vi "Movement (SubVI).vi"(4 "Speed":dbl format="%.2f", 5 "Reset":bool, 6 "Acc":dbl format="%.2f", 8 "Goal P":i32, 9 "Goal Y":dbl format="%.2f", 10 "Goal X":dbl format="%.2f") -> (0 "Vp":dbl, 1 "Vy":dbl, 2 "Vx":dbl, 3 "Reach?":bool)   [LabVIEW 2017]
uses:
  Projects/Auto control/Global 1.vi
  Projects/Auto control/Inputs.vi
  Projects/Auto control/Outputs.vi
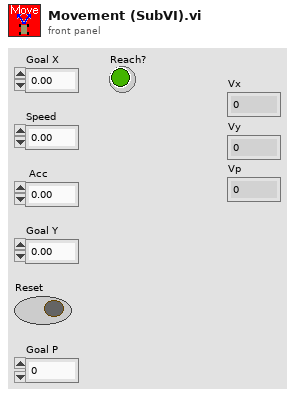
[diagram p1: front panel]
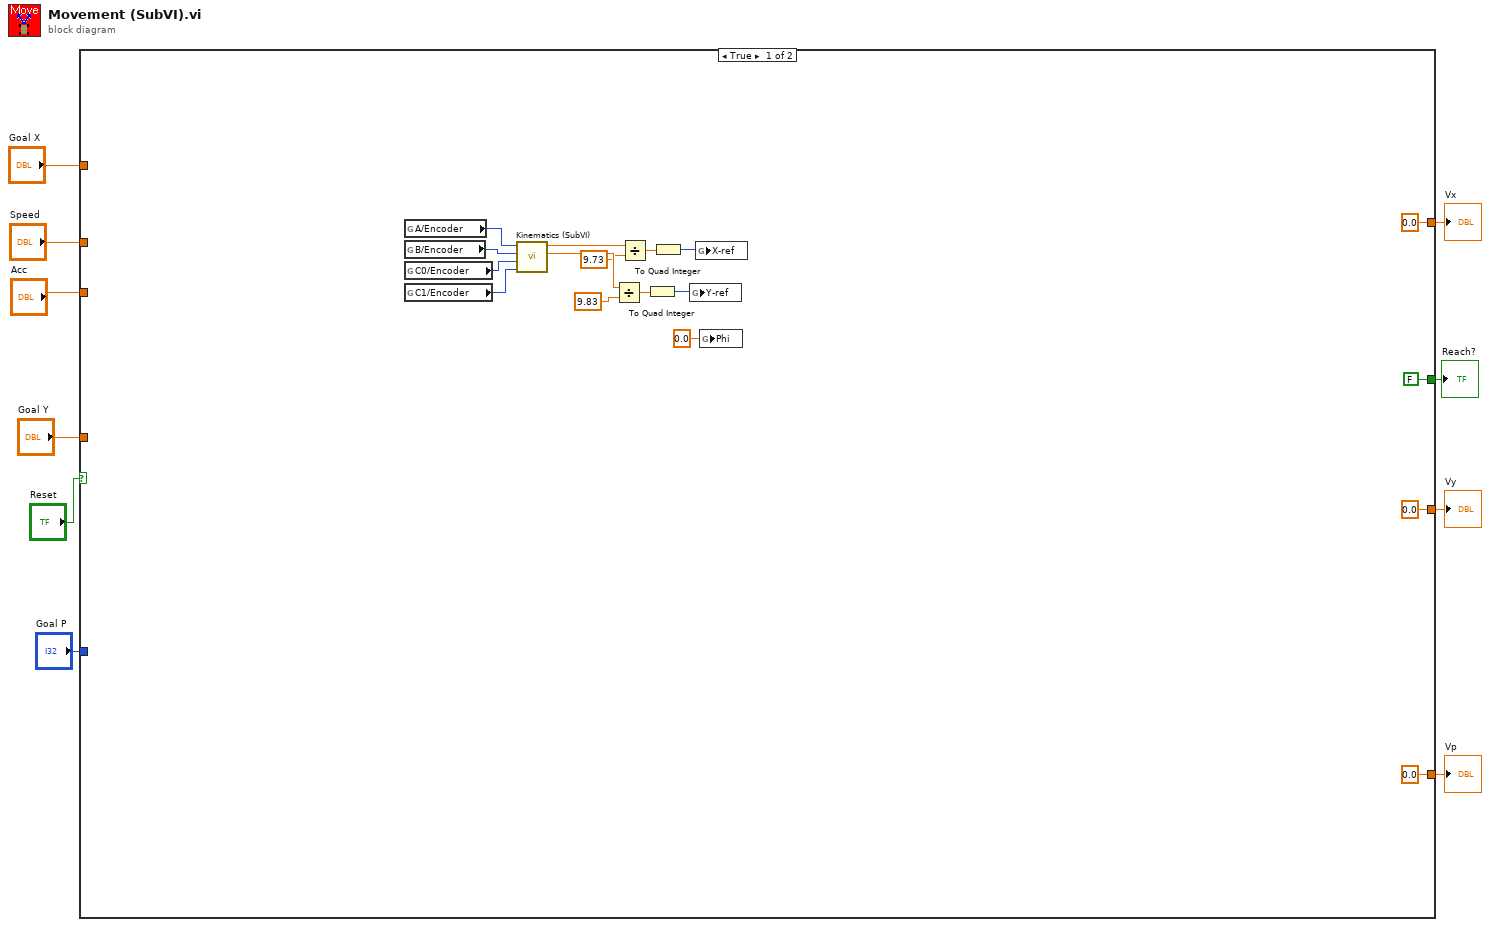
[diagram p0: block diagram]
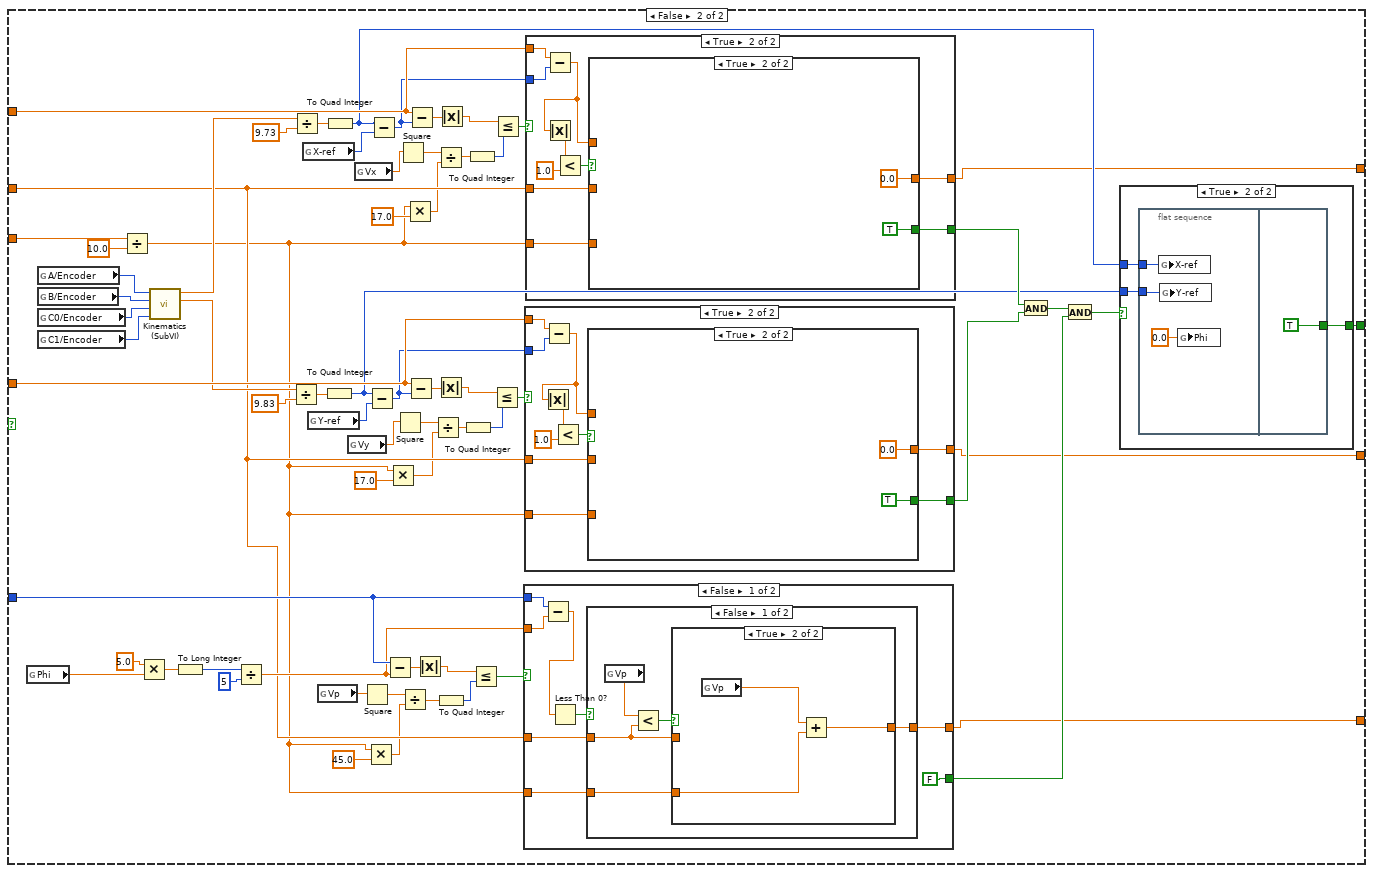
[diagram p2: hidden frame]
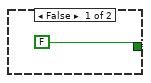
[diagram p3: hidden frame]
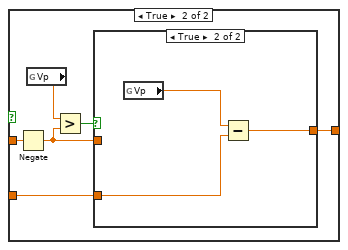
[diagram p5: hidden frame]
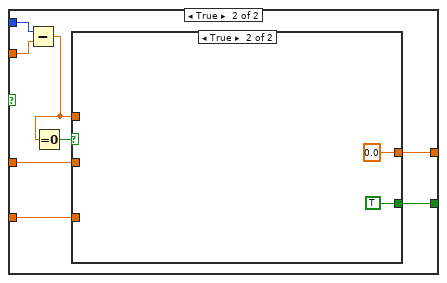
[diagram p7: hidden frame]
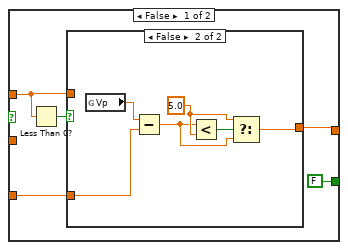
[diagram p8: hidden frame]
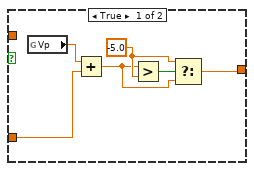
[diagram p9: hidden frame]
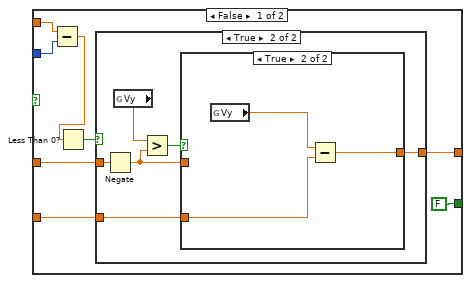
[diagram p10: hidden frame]
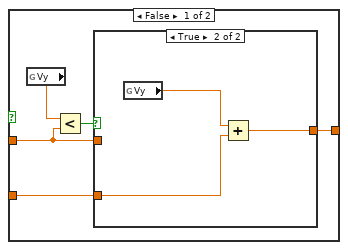
[diagram p11: hidden frame]
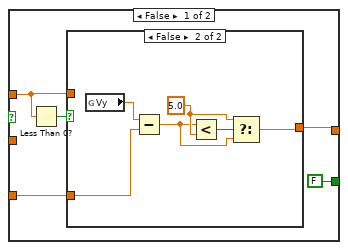
[diagram p14: hidden frame]
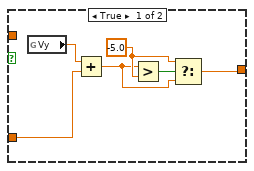
[diagram p15: hidden frame]
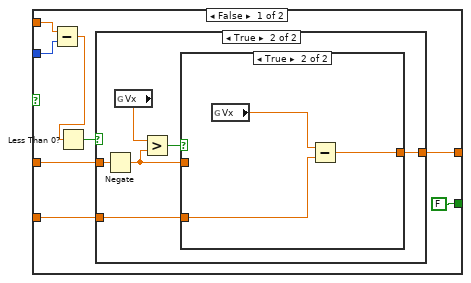
[diagram p16: hidden frame]
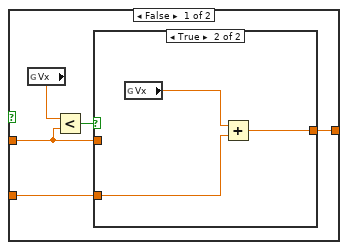
[diagram p17: hidden frame]
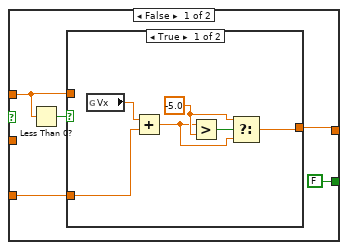
[diagram p20: hidden frame]
diagram:
  n1 = case shown="True" "Reset" {
    tunnel: "Acc" -> [_ w88]
    tunnel: "Goal X" -> [_ w86]
    tunnel: "Goal Y" -> [_ w79]
    tunnel: [FALSE ("Reach?") w71] -> w7
    tunnel: "Goal P" -> [_ w58]
    tunnel: "Speed" -> [_ w45]
    tunnel: [0.0 ("Speed") w44] -> w3
    tunnel: [0.0 ("Speed") w42] -> w2
    tunnel: [0.0 ("Speed") w43] -> w1
    frame True {
      n2 = global read "Inputs.vi" "A/Encoder"() -> (w26:i32)
      n3 = global read "Inputs.vi" "B/Encoder"() -> (w25:i32)
      n4 = global read "Inputs.vi" "C0/Encoder"() -> (w24:i32)
      n5 = global read "Inputs.vi" "C1/Encoder"() -> (w23:i32)
      n6 = call "Kinematics (SubVI).vi"("Forward Left"=w26, "Forward Right"=w25, "Back Left"=w24, "Back Right"=w23) -> ("X"=w15:dbl, "Y"=w19:dbl)  [unwired: 5 in]
      n7 = Divide(x=w19, y=9.83) -> (x/y=w21:dbl)
      n8 = Divide(x=w15, y=9.73) -> (x/y=w17:dbl)
      n9 = To Quad Integer(1:w21) -> (0:w20:i64)
      n10 = To Quad Integer(1:w17) -> (0:w16:i64)
      n11 = global write "Global 1.vi" "Y-ref"(w20) -> ()
      n12 = global write "Global 1.vi" "X-ref"(w16) -> ()
      n13 = global write "Global 1.vi" "Phi"(0.0 ("Phi")) -> ()
    }
    frame False {
      n14 = global read "Global 1.vi" "Phi"() -> (w56:dbl)
      n15 = global read "Inputs.vi" "A/Encoder"() -> (w54:i32)
      n16 = global read "Inputs.vi" "B/Encoder"() -> (w53:i32)
      n17 = global read "Inputs.vi" "C0/Encoder"() -> (w52:i32)
      n18 = global read "Inputs.vi" "C1/Encoder"() -> (w51:i32)
      n19 = Divide(x=w88, y=10.0) -> (x/y=w31:dbl)
      n20 = Multiply(x=5.0, y=w56) -> (x*y=w62:dbl)
      n21 = call "Kinematics (SubVI).vi"("Forward Left"=w54, "Forward Right"=w53, "Back Left"=w52, "Back Right"=w51) -> ("X"=w50:dbl, "Y"=w49:dbl)  [unwired: 5 in]
      n22 = To Long Integer(number=w62) -> (32bit integer=w64:i32)
      n23 = Divide(x=w64, y=5) -> (x/y=w57:dbl)
      n24 = Divide(x=w49, y=9.83) -> (x/y=w78:dbl)
      n25 = Divide(x=w50, y=9.73) -> (x/y=w85:dbl)
      n26 = global read "Global 1.vi" "X-ref"() -> (w70:i64)
      n27 = global read "Global 1.vi" "Y-ref"() -> (w69:i64)
      n28 = global read "Outputs.vi" "Vp"() -> (w28:dbl)
      n29 = To Quad Integer(1:w78) -> (0:w66:i64)
      n30 = To Quad Integer(1:w85) -> (0:w65:i64)
      n31 = global read "Outputs.vi" "Vy"() -> (w46:dbl)
      n32 = global read "Outputs.vi" "Vx"() -> (w47:dbl)
      n33 = Square(x=w28) -> (x^2=w48:dbl)
      n34 = Multiply(x=w31, y=45.0) -> (x*y=w32:dbl)
      n35 = Subtract(x=w66, y=w69) -> (x-y=w68:i64)
      n36 = Subtract(x=w65, y=w70) -> (x-y=w67:i64)
      n37 = Subtract(x=w58, y=w57) -> (x-y=w60:dbl)
      n38 = Multiply(x=w31, y=17.0) -> (x*y=w36:dbl)
      n39 = Square(x=w46) -> (x^2=w80:dbl)
      n40 = Square(x=w47) -> (x^2=w87:dbl)
      n41 = Divide(x=w48, y=w32) -> (x/y=w30:dbl)
      n42 = Multiply(x=w31, y=17.0) -> (x*y=w34:dbl)
      n43 = Subtract(x=w79, y=w68) -> (x-y=w82:dbl)
      n44 = Subtract(x=w86, y=w67) -> (x-y=w91:dbl)
      n45 = Absolute Value(x=w60) -> (abs(x)=w59:dbl)
      n46 = Divide(x=w80, y=w36) -> (x/y=w39:dbl)
      n47 = Divide(x=w87, y=w34) -> (x/y=w41:dbl)
      n48 = Absolute Value(x=w82) -> (abs(x)=w81:dbl)
      n49 = To Quad Integer(1:w30) -> (0:w29:i64)
      n50 = Absolute Value(x=w91) -> (abs(x)=w90:dbl)
      n51 = To Quad Integer(1:w39) -> (0:w38:i64)
      n52 = To Quad Integer(1:w41) -> (0:w40:i64)
      n53 = Less Or Equal?(x=w59, y=w29) -> (x <= y?=w55:bool)
      n54 = Less Or Equal?(x=w81, y=w38) -> (x <= y?=w77:bool)
      n55 = Less Or Equal?(x=w90, y=w40) -> (x <= y?=w84:bool)
      n56 = case shown="False" w55 {
        tunnel: [w107 w134] -> w43
        tunnel: w45 -> [w108 w135]
        tunnel: w31 -> [w103 w128]
        tunnel: [FALSE ("Boolean") w130] -> w73
        tunnel: w58 -> [w104 w132]
        tunnel: w57 -> [w105 w133]
        frame False {
          n57 = Subtract(x=w104, y=w105) -> (x-y=w101:dbl)
          n58 = Less Than 0?(x=w101) -> (x < 0?=w102:bool)
          n59 = case shown="False" w102 {
            tunnel: w108 -> [w109 w118]
            tunnel: w103 -> [w113 w123]
            tunnel: [w110 w120] -> w107
            frame False {
              n60 = global read "Outputs.vi" "Vp"() -> (w111:dbl)
              n61 = Less?(x=w111, y=w109) -> (x < y?=w112:bool)
              n62 = case shown="True" w112 {
                tunnel: w113 -> [_ w115]
                tunnel: [w114 w117] -> w110
                tunnel: w109 -> [w114 _]
                frame False {
                }
                frame True {
                  n63 = global read "Outputs.vi" "Vp"() -> (w116:dbl)
                  n64 = Add(x=w116, y=w115) -> (x+y=w117:dbl)
                }
              }
            }
            frame True {
              n65 = Negate(x=w118) -> (-x=w119:dbl)
              n66 = global read "Outputs.vi" "Vp"() -> (w121:dbl)
              n67 = Greater?(x=w121, y=w119) -> (0:w122:bool)
              n68 = case shown="True" w122 {
                tunnel: w123 -> [_ w125]
                tunnel: [w124 w127] -> w120
                tunnel: w119 -> [w124 _]
                frame False {
                }
                frame True {
                  n69 = global read "Outputs.vi" "Vp"() -> (w126:dbl)
                  n70 = Subtract(x=w126, y=w125) -> (x-y=w127:dbl)
                }
              }
            }
          }
        }
        frame True {
          n71 = Subtract(x=w132, y=w133) -> (x-y=w129:dbl)
          n72 = Equal To 0?(x=w129) -> (x = 0?=w131:bool)
          n73 = case shown="True" w131 {
            tunnel: w135 -> [_ _]
            tunnel: [w136 0.0 ("Speed")] -> w134
            tunnel: [FALSE ("Boolean") TRUE ("Boolean")] -> w130
            tunnel: w129 -> [w138 _]
            tunnel: w128 -> [w137 _]
            frame False {
              n74 = Less Than 0?(x=w138) -> (x < 0?=w139:bool)
              n75 = case shown="False" w139 {
                tunnel: w138 -> [_ _]
                tunnel: w137 -> [w145 w151]
                tunnel: [w141 w147] -> w136
                frame True {
                  w143 = -5.0 ("y")
                  n76 = global read "Outputs.vi" "Vp"() -> (w146:dbl)
                  n77 = Add(x=w146, y=w145) -> (x+y=w142:dbl)
                  n78 = Greater?(x=w142, y=w143) -> (0:w144:bool)
                  n79 = Select(t=w143, s=w144, f=w142) -> (s? t:f=w141:dbl)
                }
                frame False {
                  w149 = 5.0 ("y")
                  n80 = global read "Outputs.vi" "Vp"() -> (w152:dbl)
                  n81 = Subtract(x=w152, y=w151) -> (x-y=w148:dbl)
                  n82 = Less?(x=w148, y=w149) -> (x < y?=w150:bool)
                  n83 = Select(t=w149, s=w150, f=w148) -> (s? t:f=w147:dbl)
                }
              }
            }
            frame True {
            }
          }
        }
      }
      n84 = case shown="True" w77 {
        tunnel: [w161 w190] -> w42
        tunnel: w45 -> [w162 w191]
        tunnel: w31 -> [w155 w186]
        tunnel: [FALSE ("Boolean") w187] -> w76
        tunnel: w79 -> [w158 w188]
        tunnel: w68 -> [w159 w189]
        frame False {
          n85 = Subtract(x=w158, y=w159) -> (x-y=w156:dbl)
          n86 = Less Than 0?(x=w156) -> (x < 0?=w157:bool)
          n87 = case shown="True" w157 {
            tunnel: w162 -> [w163 w172]
            tunnel: w155 -> [w167 w177]
            tunnel: [w164 w174] -> w161
            frame False {
              n88 = global read "Outputs.vi" "Vy"() -> (w165:dbl)
              n89 = Less?(x=w165, y=w163) -> (x < y?=w166:bool)
              n90 = case shown="True" w166 {
                tunnel: w167 -> [_ w169]
                tunnel: [w168 w171] -> w164
                tunnel: w163 -> [w168 _]
                frame False {
                }
                frame True {
                  n91 = global read "Outputs.vi" "Vy"() -> (w170:dbl)
                  n92 = Add(x=w170, y=w169) -> (x+y=w171:dbl)
                }
              }
            }
            frame True {
              n93 = Negate(x=w172) -> (-x=w173:dbl)
              n94 = global read "Outputs.vi" "Vy"() -> (w175:dbl)
              n95 = Greater?(x=w175, y=w173) -> (0:w176:bool)
              n96 = case shown="True" w176 {
                tunnel: w177 -> [_ w179]
                tunnel: [w178 w181] -> w174
                tunnel: w173 -> [w178 _]
                frame False {
                }
                frame True {
                  n97 = global read "Outputs.vi" "Vy"() -> (w180:dbl)
                  n98 = Subtract(x=w180, y=w179) -> (x-y=w181:dbl)
                }
              }
            }
          }
        }
        frame True {
          n99 = Subtract(x=w188, y=w189) -> (x-y=w182:dbl)
          n100 = Absolute Value(x=w182) -> (abs(x)=w185:dbl)
          n101 = Less?(x=w185, y=1.0) -> (x < y?=w183:bool)
          n102 = case shown="True" w183 {
            tunnel: w191 -> [_ _]
            tunnel: [w192 0.0 ("Speed")] -> w190
            tunnel: [FALSE ("Boolean") TRUE ("Boolean")] -> w187
            tunnel: w182 -> [w194 _]
            tunnel: w186 -> [w193 _]
            frame False {
              n103 = Less Than 0?(x=w194) -> (x < 0?=w195:bool)
              n104 = case shown="False" w195 {
                tunnel: w194 -> [_ _]
                tunnel: w193 -> [w201 w207]
                tunnel: [w197 w203] -> w192
                frame True {
                  w199 = -5.0 ("y")
                  n105 = global read "Outputs.vi" "Vy"() -> (w202:dbl)
                  n106 = Add(x=w202, y=w201) -> (x+y=w198:dbl)
                  n107 = Greater?(x=w198, y=w199) -> (0:w200:bool)
                  n108 = Select(t=w199, s=w200, f=w198) -> (s? t:f=w197:dbl)
                }
                frame False {
                  w205 = 5.0 ("y")
                  n109 = global read "Outputs.vi" "Vy"() -> (w208:dbl)
                  n110 = Subtract(x=w208, y=w207) -> (x-y=w204:dbl)
                  n111 = Less?(x=w204, y=w205) -> (x < y?=w206:bool)
                  n112 = Select(t=w205, s=w206, f=w204) -> (s? t:f=w203:dbl)
                }
              }
            }
            frame True {
            }
          }
        }
      }
      n113 = case shown="True" w84 {
        tunnel: [w217 w246] -> w44
        tunnel: w45 -> [w218 w247]
        tunnel: w31 -> [w211 w242]
        tunnel: [FALSE ("Boolean") w243] -> w75
        tunnel: w86 -> [w214 w244]
        tunnel: w67 -> [w215 w245]
        frame False {
          n114 = Subtract(x=w214, y=w215) -> (x-y=w212:dbl)
          n115 = Less Than 0?(x=w212) -> (x < 0?=w213:bool)
          n116 = case shown="True" w213 {
            tunnel: w218 -> [w219 w228]
            tunnel: w211 -> [w223 w233]
            tunnel: [w220 w230] -> w217
            frame False {
              n117 = global read "Outputs.vi" "Vx"() -> (w221:dbl)
              n118 = Less?(x=w221, y=w219) -> (x < y?=w222:bool)
              n119 = case shown="True" w222 {
                tunnel: w223 -> [_ w225]
                tunnel: [w224 w227] -> w220
                tunnel: w219 -> [w224 _]
                frame False {
                }
                frame True {
                  n120 = global read "Outputs.vi" "Vx"() -> (w226:dbl)
                  n121 = Add(x=w226, y=w225) -> (x+y=w227:dbl)
                }
              }
            }
            frame True {
              n122 = Negate(x=w228) -> (-x=w229:dbl)
              n123 = global read "Outputs.vi" "Vx"() -> (w231:dbl)
              n124 = Greater?(x=w231, y=w229) -> (0:w232:bool)
              n125 = case shown="True" w232 {
                tunnel: w233 -> [_ w235]
                tunnel: [w234 w237] -> w230
                tunnel: w229 -> [w234 _]
                frame False {
                }
                frame True {
                  n126 = global read "Outputs.vi" "Vx"() -> (w236:dbl)
                  n127 = Subtract(x=w236, y=w235) -> (x-y=w237:dbl)
                }
              }
            }
          }
        }
        frame True {
          n128 = Subtract(x=w244, y=w245) -> (x-y=w240:dbl)
          n129 = Absolute Value(x=w240) -> (abs(x)=w239:dbl)
          n130 = Less?(x=w239, y=1.0) -> (x < y?=w241:bool)
          n131 = case shown="True" w241 {
            tunnel: w247 -> [_ _]
            tunnel: [w248 0.0 ("Speed")] -> w246
            tunnel: [FALSE ("Boolean") TRUE ("Boolean")] -> w243
            tunnel: w240 -> [w250 _]
            tunnel: w242 -> [w249 _]
            frame False {
              n132 = Less Than 0?(x=w250) -> (x < 0?=w251:bool)
              n133 = case shown="True" w251 {
                tunnel: w250 -> [_ _]
                tunnel: w249 -> [w257 w263]
                tunnel: [w253 w259] -> w248
                frame True {
                  w255 = -5.0 ("y")
                  n134 = global read "Outputs.vi" "Vx"() -> (w258:dbl)
                  n135 = Add(x=w258, y=w257) -> (x+y=w254:dbl)
                  n136 = Greater?(x=w254, y=w255) -> (0:w256:bool)
                  n137 = Select(t=w255, s=w256, f=w254) -> (s? t:f=w253:dbl)
                }
                frame False {
                  w261 = 5.0 ("y")
                  n138 = global read "Outputs.vi" "Vx"() -> (w264:dbl)
                  n139 = Subtract(x=w264, y=w263) -> (x-y=w260:dbl)
                  n140 = Less?(x=w260, y=w261) -> (x < y?=w262:bool)
                  n141 = Select(t=w261, s=w262, f=w260) -> (s? t:f=w259:dbl)
                }
              }
            }
            frame True {
            }
          }
        }
      }
      n142 = And(x=w75, y=w76) -> (x .and. y?=w74:bool)
      n143 = And(x=w74, y=w73) -> (x .and. y?=w72:bool)
      n144 = case shown="True" w72 {
        tunnel: [FALSE ("Reach?") w96] -> w71
        tunnel: w66 -> [_ w95]
        tunnel: w65 -> [_ w94]
        frame False {
        }
        frame True {
          n145 = flat-sequence {
            tunnel: w95 -> [w99]
            tunnel: w94 -> [w98]
            tunnel: [TRUE ("Reach?")] -> w96
            frame #0 {
              n146 = global write "Global 1.vi" "X-ref"(w98) -> ()
              n147 = global write "Global 1.vi" "Y-ref"(w99) -> ()
              n148 = global write "Global 1.vi" "Phi"(0.0 ("Phi")) -> ()
            }
            frame #1 {
            }
          }
        }
      }
    }
  }
  "Reach?" <- w7
  "Vx" <- w3
  "Vy" <- w2
  "Vp" <- w1
